vi "FITS_ReadImgSGL.vi"(8 "error in":errorcluster, 10 "ref":u64) -> (0 "error out":errorcluster, 2 "Img Data":sgl[](array[numeric]) format="%.2f")   [LabVIEW 2016]
uses:
  usr/local/lib/libfits.so
panel:
  in  "Memory":sgl[](array[numeric]) format="%.2f"
  out "result":i32
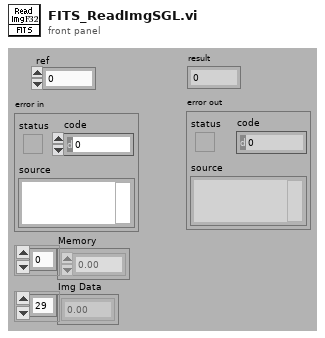
[diagram p1: front panel]
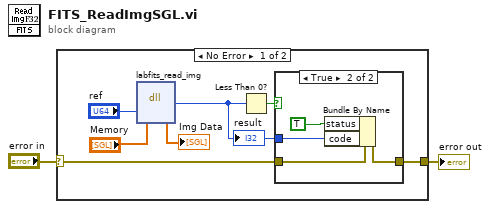
[diagram p0: block diagram]
diagram:
  n1 = case shown="No Error" "error in" {
    selector: "error in" -> [w8 w15]
    tunnel: [w7 w15] -> w1
    frame No Error {
      n2 = dll-call lib="usr/local/lib/libfits.so" fn="labfits_read_img"("ref"="ref", "bufData"="Memory") -> ("return type"=w6:i32, "bufData"=→"Img Data":sgl[])  [unwired: 4 in, 2 out]
      "result" <- w6
      n3 = Less Than 0?(x=w6) -> (x < 0?=w9:bool)
      n4 = case shown="True" w9 {
        tunnel: w8 -> [w10 w12]
        tunnel: [w10 w11] -> w7
        tunnel: w6 -> [_ w13]
        frame False {
        }
        frame True {
          n5 = Bundle By Name(cluster=w12, "status"=TRUE, "code"=w13) -> (w11:errorcluster)
        }
      }
    }
    frame Error {
    }
  }
  "error out" <- w1
